vi "subvi_encoder_tick_to_pos.vi"(0 "Velocity Interval (uSec)":u32=1000, 1 "Raw Tick":i32, 5 "Waited?'":bool, 7 "Tick Count(uSec)'":u32, 9 "p'":i32, 11 "Time Count":u32, 12 "a'":i32, 13 "v'":i32) -> (2 "Waited?":bool, 3 "Tick Count(uSec)":u32, 4 "p":i32, 6 "v":i32, 8 "a":i32)   [LabVIEW 2019]
uses:
  <vilib>/rvi/Arithmetic/AddSubMult/XNode/nirviSatArithmetic.xnode
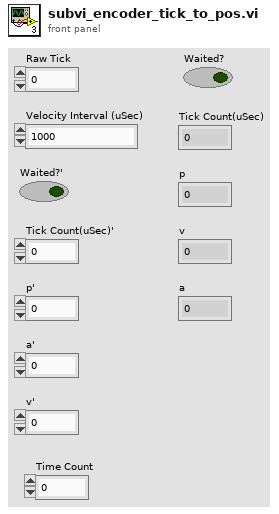
[diagram p1: front panel]
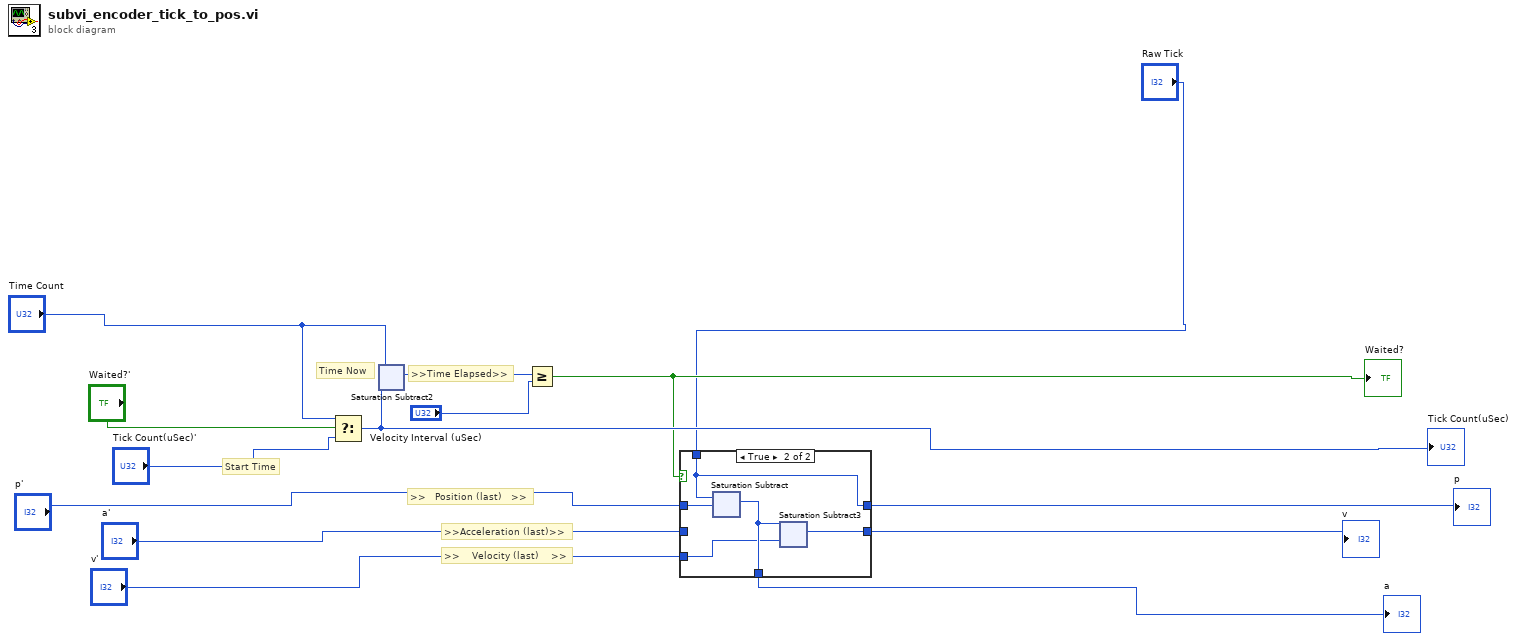
[diagram p0: block diagram]
diagram:
  # ">>Acceleration (last)>>"
  # "Start Time"
  # ">>    Velocity (last)    >>"
  # ">>   Position (last)   >>"
  # "Time Now"
  # ">>Time Elapsed>>"
  n1 = Select(t="Time Count", s="Waited?'", f="Tick Count(uSec)'") -> (s? t:f=w13:u32)
  "Tick Count(uSec)" <- w13
  n2 = xnode ("Saturation Subtract2")("x"="Time Count", "y"=w13) -> ("x-y"=w3:u32)
  n3 = Greater Or Equal?(x=w3, y="Velocity Interval (uSec)") -> (x >= y?=w11:bool)
  "Waited?" <- w11
  n4 = case shown="True" w11 {
    tunnel: "Raw Tick" -> [_ w18]
    tunnel: "p'" -> [w15 w22]
    tunnel: [w17 w21] -> w4
    tunnel: "v'" -> [w17 w20]
    tunnel: [w16 w19] -> w6
    tunnel: "a'" -> [w16 _]
    tunnel: [w15 w18] -> w8
    frame False {
    }
    frame True {
      n5 = xnode ("Saturation Subtract")("x"=w18, "y"=w22) -> ("x-y"=w21:i32)
      n6 = xnode ("Saturation Subtract3")("x"=w21, "y"=w20) -> ("x-y"=w19:i32)
    }
  }
  "p" <- w8
  "v" <- w6
  "a" <- w4
